vi "save_data (SubVI).vi"(10 "Filename":path, 11 "data tasks":T2) -> (2 "output data tasks":T1, 3 "Output data":dbl[][](array[numeric]))   [LabVIEW 2014]
uses:
  <vilib>/addons/h5labview2/file/H5Fmode.ctl
  <vilib>/DAQmx/read.llb/DAQmx Read (Analog 2D DBL NChan NSamp).vi
  <vilib>/addons/h5labview2/base/lib_path.vi
  <vilib>/addons/h5labview2/base/H5Equery.vi
  <vilib>/addons/h5labview2/dataset/H5Dwrite.llb/H5Dwrite.xnode
  <vilib>/addons/h5labview2/attrib/H5Awrite.llb/H5Awrite.xnode
  <vilib>/addons/h5labview2/base/hid_t.ctl
  <vilib>/addons/h5labview2/file/H5F.lvlib
  <vilib>/addons/h5labview2/group/H5G.lvlib
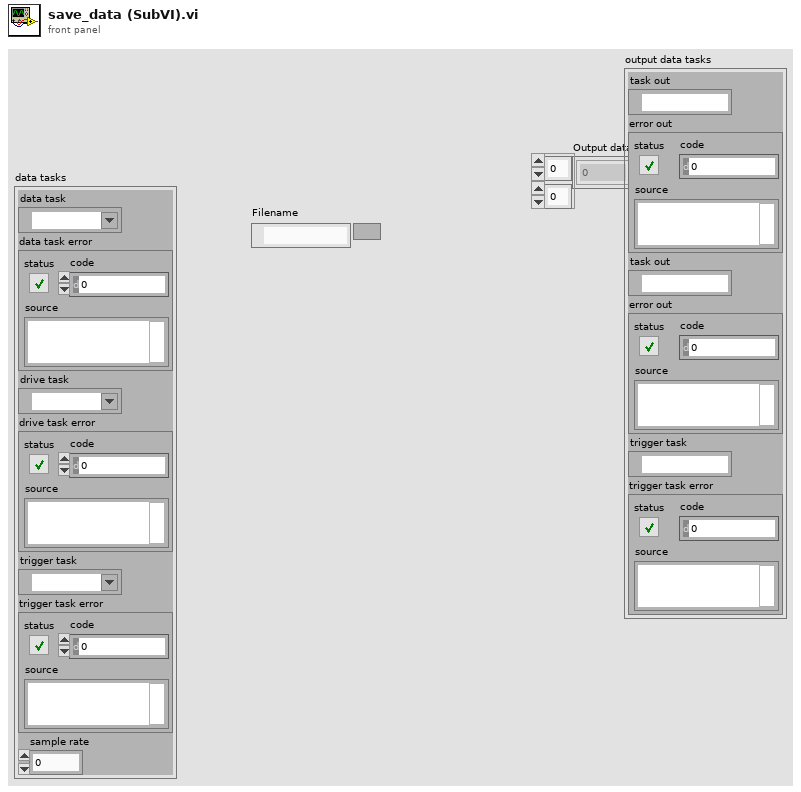
[diagram p1: front panel]
types:
  T1 = cluster{"task out":refnum<k21>, "error out":errorcluster, "task out":refnum<k21>, "error out":errorcluster, "trigger task":refnum<k21>, "trigger task error":errorcluster}
  T2 = cluster{"data task":refnum<k21>, "data task error":errorcluster, "drive task":refnum<k21>, "drive task error":errorcluster, "trigger task":refnum<k21>, "trigger task error":errorcluster, "sample rate":dbl}
  T3 = typedef "H5F.lvlib/H5Fmode.ctl" = enum16{"read-only", "read-write", "overwrite", "create new", "open or create"}
  T4 = typedef "hid_t.ctl" = i32
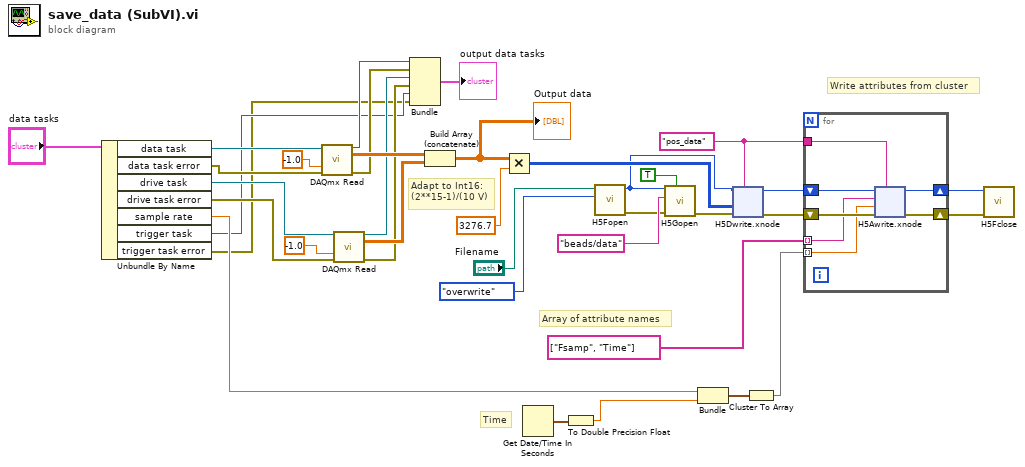
[diagram p0: block diagram]
diagram:
  w27 = "pos_data" ("dataset name")
  # "Time"
  # "Array of attribute names"
  # "Write attributes from cluster"
  # "Adapt to Int16: \n(2**15-1)/(10 V)"
  n1 = Unbundle By Name("data tasks") -> ("data task"=w36:refnum<k21>, "data task error"=w35:errorcluster, "drive task"=w33:refnum<k21>, "drive task error"=w32:errorcluster, "sample rate"=w20:dbl, "trigger task"=w3:refnum<k21>, "trigger task error"=w2:errorcluster)
  n2 = call-poly <vilib>:"DAQmx Read.vi"("task/channels in"=w36, "timeout"=-1.0, "error in"=w35) -> ("task out"=w7:refnum<k21>, "data"=w30:dbl[][], "error out"=w6:errorcluster)  [unwired: 10 in]
  n3 = call-poly <vilib>:"DAQmx Read.vi"("task/channels in"=w33, "timeout"=-1.0, "error in"=w32) -> ("task out"=w5:refnum<k21>, "data"=w29:dbl[][], "error out"=w4:errorcluster)  [unwired: 10 in]
  n4 = Bundle("task out"=w7, "error out"=w6, "task out"=w5, "error out"=w4, "trigger task"=w3, "trigger task error"=w2) -> (→"output data tasks":T1)  [unwired: 1 in]
  n5 = Build Array (concatenate)(w30, w29) -> (w11:dbl[][])
  "Output data" <- w11
  n6 = Multiply(x=w11, y=3276.7) -> (x*y=w24:i16[][])
  n7 = Get Date/Time In Seconds() -> (seconds since 1Jan1904=w21:timestamp)
  n8 = To Double Precision Float(number=w21) -> (double precision float=w18:dbl)
  n9 = call <vilib>:"H5Fopen.vi"("mode (read-only)"=H5Fmode."overwrite", "path"="Filename") -> ("error out"=w12:errorcluster, "ref out"=w9:T4)  [unwired: 8 in]
  n10 = call <vilib>:"H5Gopen.vi"("create? (F)"=TRUE, "error in (no error)"=w12, "name"="beads/data", "ref in"=w9) -> ("error out"=w23:errorcluster)  [unwired: 6 in, 1 out]
  n11 = Bundle("sample rate"=w20, w18) -> (w17:cluster{"sample rate":dbl, dbl})  [unwired: 1 in]
  n12 = xnode "H5Dwrite.xnode"("dataset name"=w27, "error in (no error)"=w23, "data"=w24, "ref in"=w9) -> ("error out"=w22:errorcluster, "ref out"=w8:i32)  [unwired: 3 in, 1 out]
  n13 = Cluster To Array(cluster=w17) -> (array=w16:dbl[])
  n14 = for {
    tunnel: w27 -> [w44]
    shift-right: [w42] -> w15
    shift-left: w8 -> [w38]
    shift-right: [w41] -> w14
    shift-left: w22 -> [w43]
    tunnel: string[] ["Fsamp", "Time"] -> [w40] mode=indexing
    tunnel: w16 -> [w39] mode=indexing
    n15 = xnode "H5Awrite.xnode"("object name"=w44, "error in (no error)"=w43, "data"=w39, "attrib name"=w40, "ref in"=w38) -> ("error out"=w41:errorcluster, "ref out"=w42:T4)  [unwired: 2 in, 1 out]
  }
  n16 = call <vilib>:"H5Fclose.vi"("error in (no error)"=w14, "ref"=w15) -> ()  [unwired: 9 in, 1 out]
